vi "Read Last Known State.vi"(8 "error in (no error)":errorcluster, 11 "FP-TC-Shared.lvclass":refnum<class "FP-TC-Shared.lvclass">) -> (0 "error out":errorcluster, 3 "FP-TC-Shared.lvclass":refnum<class "FP-TC-Shared.lvclass">)   [LabVIEW 2019, in "FP-TC-Shared.lvclass"]
uses:
  FP-TC-Shared.lvclass
  FP-TC-Shared.lvclass/FP-TC-Shared.ctl
  <userlib>/LevyLab/Instrument Framework/SMOs/Configuration/Configuration.lvclass/Configuration.ctl
  <userlib>/LevyLab/Instrument Framework/SMOs/Configuration/Configuration.lvclass
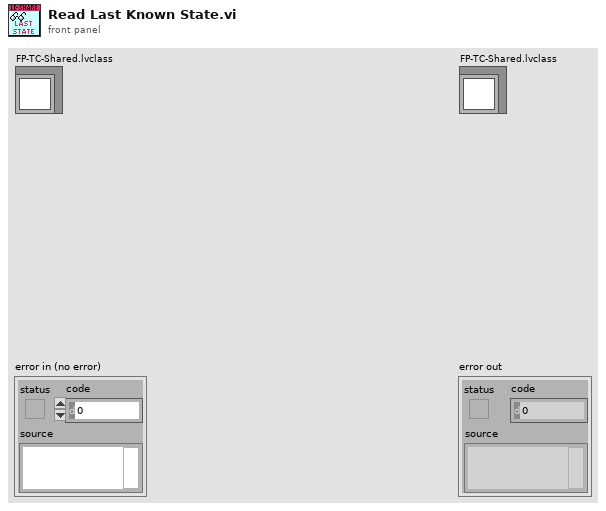
[diagram p1: front panel]
types:
  T1 = typedef "FP-TC-Shared.lvclass/LC Type--Enum.ctl" = enum16{"CF.TC", "CF.TC.Z", "CF.FP", "MNK.TC", "MNK.TC.Z", "MNK.FP"}
  T2 = cluster{"Application":enum16{"TC", "FP"}, "LC Type":T1}
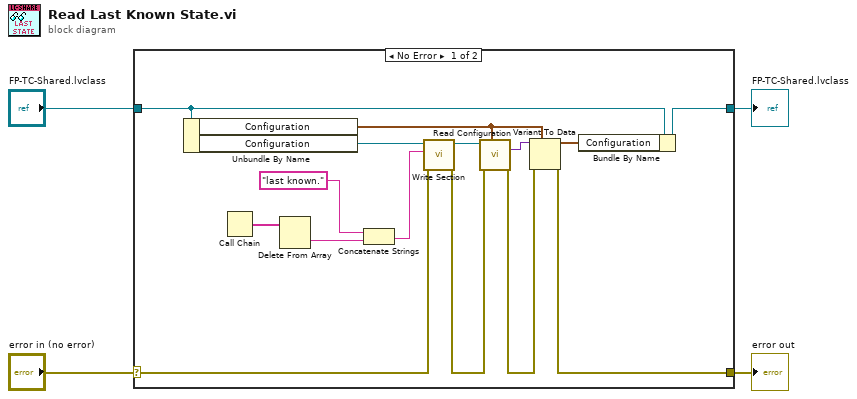
[diagram p0: block diagram]
diagram:
  n1 = case shown="No Error" "error in (no error)" {
    selector: "error in (no error)" -> [w11 w21]
    tunnel: [w5 w21] -> w3
    tunnel: [w7 w20] -> w1
    tunnel: "FP-TC-Shared.lvclass" -> [w6 w20]
    frame No Error {
      n2 = Unbundle By Name(w6) -> ("Configuration"=w12:T2, "Configuration"=w16:refnum<class "Configuration.lvclass">)
      n3 = Call Chain() -> (call chain=w19:string[])
      n4 = Delete From Array(array=w19) -> (deleted portion=w17:string)  [unwired: 2 in, 1 out]
      n5 = Concatenate Strings("last known.", w17) -> (w15:string)
      n6 = call <userlib>:"Write Section.vi"("error in (no error)"=w11, "Section"=w15, "Configuration in"=w16) -> ("error out"=w10:errorcluster, "Configuration out"=w14:refnum<class "Configuration.lvclass">)  [unwired: 7 in]
      n7 = call <userlib>:"Read Configuration.vi"("INI Fomatted Cluster Type"=w12, "error in (no error)"=w10, "Configuration in"=w14) -> ("error out"=w9:errorcluster, "Configuration"=w13:variant)  [unwired: 6 in, 1 out]
      n8 = Variant To Data(error in=w9, type=w12, Variant=w13) -> (data=w8:T2, error out=w5:errorcluster)
      n9 = Bundle By Name(cluster=w6, "Configuration"=w8) -> (w7:refnum<class "FP-TC-Shared.lvclass">)
    }
    frame Error {
    }
  }
  "error out" <- w3
  "FP-TC-Shared.lvclass" <- w1
